vi "CleanUpDiagram.vi"(0 "__args":cluster{"targetVi":string}) -> (1 "__return":i32, 2 "__errStatus":bool, 3 "__errCode":i32, 4 "__errSource":string)   [LabVIEW 2013]
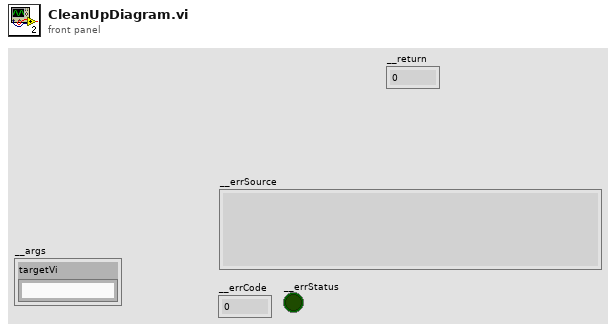
[diagram p1: front panel]
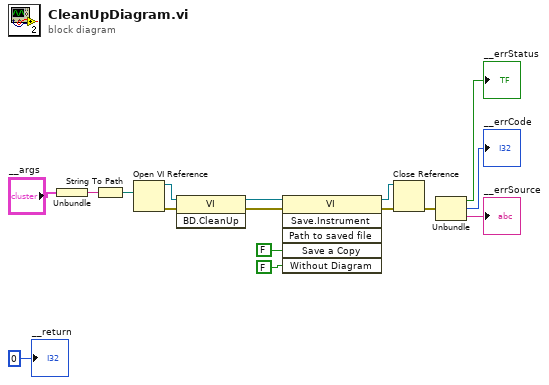
[diagram p0: block diagram]
diagram:
  n1 = Unbundle("__args") -> ("targetVi"=w12:string)
  n2 = String To Path(string=w12) -> (path=w11:path)
  n3 = Open VI Reference(vi path=w11) -> (vi reference=w4:refnum<vi>, error out=w1:errorcluster)  [unwired: 5 in]
  n4 = invoke class="VI" method="BD.CleanUp"(reference=w4, error in=w1) -> (reference out=w3:refnum<vi>, error out=w2:errorcluster)  [unwired: 1 in, 1 out]
  n5 = invoke class="VI" method="Save.Instrument"(reference=w3, error in=w2, "Save a Copy"=FALSE, "Without Diagram"=FALSE) -> (reference out=w9:refnum<vi>, error out=w7:errorcluster)  [unwired: 2 in, 4 out]
  n6 = Close Reference(reference=w9, error in (no error)=w7) -> (error out=w8:errorcluster)
  n7 = Unbundle(w8) -> ("status"=→"__errStatus":bool, "code"=→"__errCode":i32, "source"=→"__errSource":string)
  "__return" <- 0
